vi "Logging.vi"   [LabVIEW 2017]
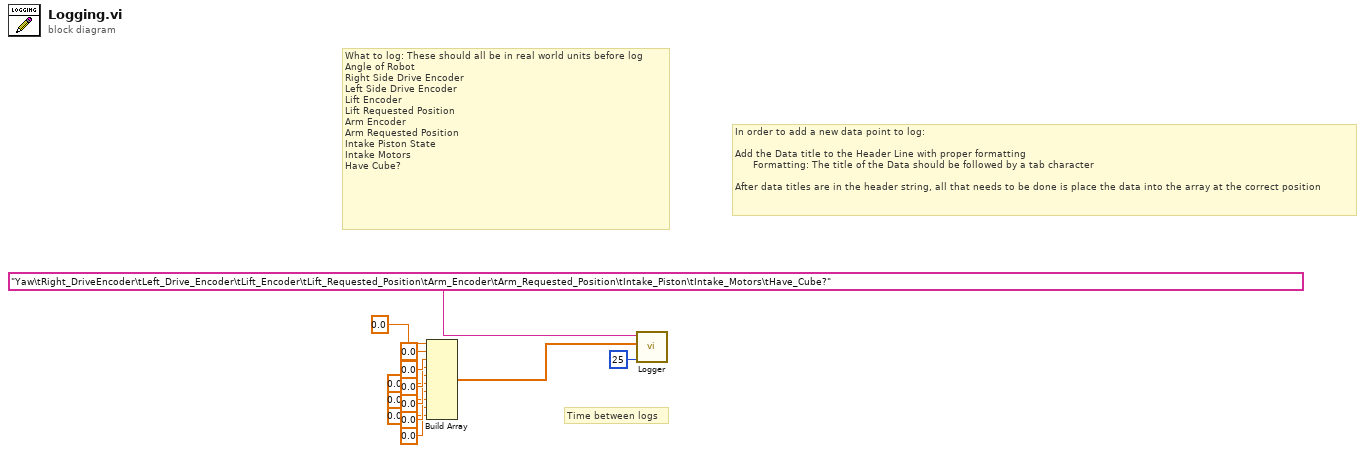
[diagram p0: block diagram]
diagram:
  # "Time between logs"
  # "In order to add a new data point to log:\n\nAdd the Data title to the Header Line with proper formatting\n      Formatting: The title of the Data should be followed by a tab character\n\nAfter data titles are in the header string, all that needs to be done is place the data into the array at the correct position"
  # "What to log: These should all be in real world units before log\nAngle of Robot\nRight Side Drive Encoder\nLeft Side Drive Encoder\nLift Encoder\nLift Requested Position\nArm Encoder\nArm Requested Position\nIntake Piston State\nIntake Motors\nHave Cube?"
  n1 = Build Array(0.0 ("element"), 0.0 ("element"), 0.0 ("element"), 0.0 ("element"), 0.0 ("element"), 0.0 ("element"), 0.0 ("element"), 0.0 ("element"), 0.0 ("element"), 0.0 ("element")) -> (w12:dbl[])
  n2 = call "Logger.vi"("Time Between Loops"=i64 25, "Data"=w12, "Header Line"="Yaw\tRight_DriveEncoder\tLeft_Drive_Encoder\tLift_Encoder\tLift_Requested_Position\tArm_Encoder\tArm_Requested_Position\tIntake_Piston\tIntake_Motors\tHave_Cube?") -> ()  [unwired: 9 in]
